vi "Main.vi"(8 "error in (no error)":errorcluster, 11 "GalvoBase in":refnum<class "ImagingModeSPIM.lvclass">) -> (0 "error out":errorcluster, 3 "component":refnum<class "ImagingModeSPIM.lvclass">)   [LabVIEW 2012, in "ImagingModeSPIM.lvclass"]
doc: "Main VI of the component."
uses:
  ImagingModeSPIM.lvclass
  Controls/waveform_enum.ctl
  ImagingModeSPIM.lvclass/ImagingModeSPIM.ctl
  <vilib>/Distrio/Murmex/InitialiseMessage/InitialiseMessage.lvclass
  <vilib>/Distrio/Murmex/TerminateMessage/TerminateMessage.lvclass
  <vilib>/Distrio/Murmex/ConfigureMessage/ConfigureMessage.lvclass
  <vilib>/Distrio/Murmex/StopMessage/StopMessage.lvclass
  <vilib>/Distrio/Murmex/StartMessage/run mode enum.ctl
  <vilib>/Distrio/Murmex/StartMessage/StartMessage.lvclass
  <vilib>/Distrio/Murmex/Murmex/update_cluster.ctl
  <vilib>/Distrio/Murmex/Murmex/Set configure at initialise.vi
  <vilib>/Distrio/Murmex/Murmex/Set VI reference.vi
  <vilib>/Distrio/Murmex/Murmex/Get ID.vi
  <vilib>/Distrio/Murmex/Murmex/Set relay start stop to observers.vi
  <vilib>/Distrio/Murmex/Murmex/Set log reference.vi
  <vilib>/Distrio/Murmex/Murmex/Set license required.vi
  <vilib>/Distrio/Murmex/StartMessage/Set run mode.vi
  <vilib>/Distrio/Murmex/Murmex/Murmex.lvclass
panel:
  in  "button::quit":bool
  in  "button:start_finite":bool
  in  "button:start_free-run":bool
  in  "button::configure":bool
  in  "Tab Control":T1(tab)
  in  "Phase 2":dbl[unit] caption="phase" min=-6.283185307179586 max=6.283185307179586 step=0.0017453292519943296
  in  "Offset 2":dbl[unit] caption="offset" min=-5.0 max=5.0 step=0.01
  in  "Amplitude 2":dbl[unit]=1.0 caption="amplitude" min=0.0 max=5.0 step=0.01
  in  "Phase 1":dbl[unit] caption="phase" min=-6.283185307179586 max=6.283185307179586 step=0.0017453292519943296
  in  "shape":T2
  in  "Offset 1":dbl[unit] caption="offset" min=-5.0 max=5.0 step=0.01
  in  "Amplitude 1":dbl[unit]=1.0 caption="amplitude" min=0.0 max=5.0 step=0.01
  in  "frame time":dbl[unit]=100.0
  in  "frames":i32=1
  in  "v lines":i32=2048 min=4 max=2048 step=4
  in  "digital pulses":i32=2 min=0 max=20 step=2
  in  "digital ratio":dbl(knob)=0.5 min=0.0 max=1.0 step=0.02 scale=0.0..1.0
  out "log":string
  in  "ID":string="spim"
  out "terminate?":bool=TRUE
  # "galvo 1"
  # "galvo 2"
  # "ImagingModeSPIM\n\nDeveloped by:\n\nMarcel van 't Hoff PhD, \nMarie Caroline Muellenbroich PhD, \nLudovico Silvestri PhD,\n   University of Florence, 2014"
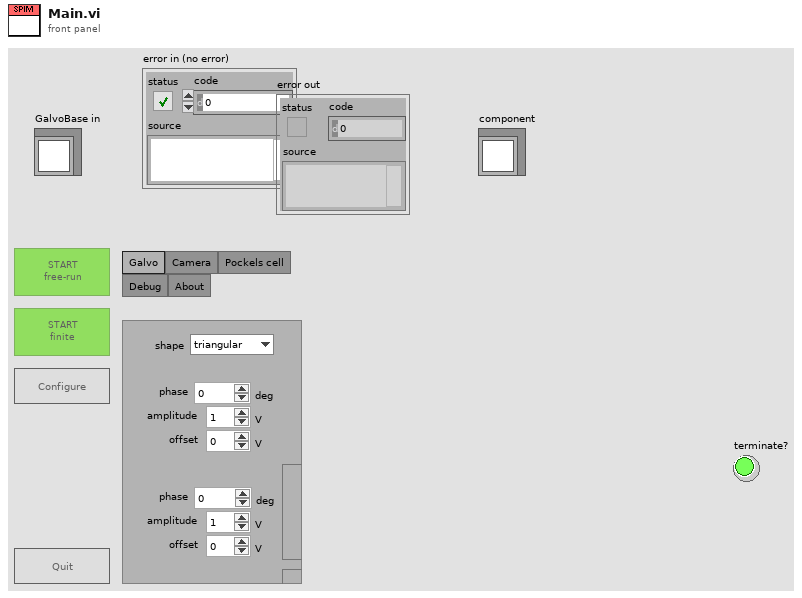
[diagram p1: front panel]
types:
  T1 = enum32{"Galvo", "Camera", "Pockels cell", "Debug", "About"}
  T2 = typedef "ImagingModeSPIM.lvclass/waveform_enum.ctl" = enum16{"triangular", "sawtooth", "sinusodial"}
  T3 = enum8{"Enabled", "Disabled", "Disabled and Grayed Out"}
  T4 = typedef "Murmex.lvlib/StartMessage.lvclass/run mode enum.ctl" = enum16{"infinite", "finite"}
  T5 = typedef "Murmex.lvlib/Murmex.lvclass/update_cluster.ctl" = cluster{"target ID":string, "key chains":string[], "values":variant[]}
  T6 = typedef "Murmex.lvlib/Murmex.lvclass/command_enum.ctl" = enum16{"null", "initialise", "reset", "terminate", "acknowledge", "update", "inspect", "inform", "proceed", "start", "stop", "fetch", "configure", "generic"}
  T7 = typedef "Murmex.lvlib/Murmex.lvclass/Event type enumerations.ctl" = enum16{"before", "after"}
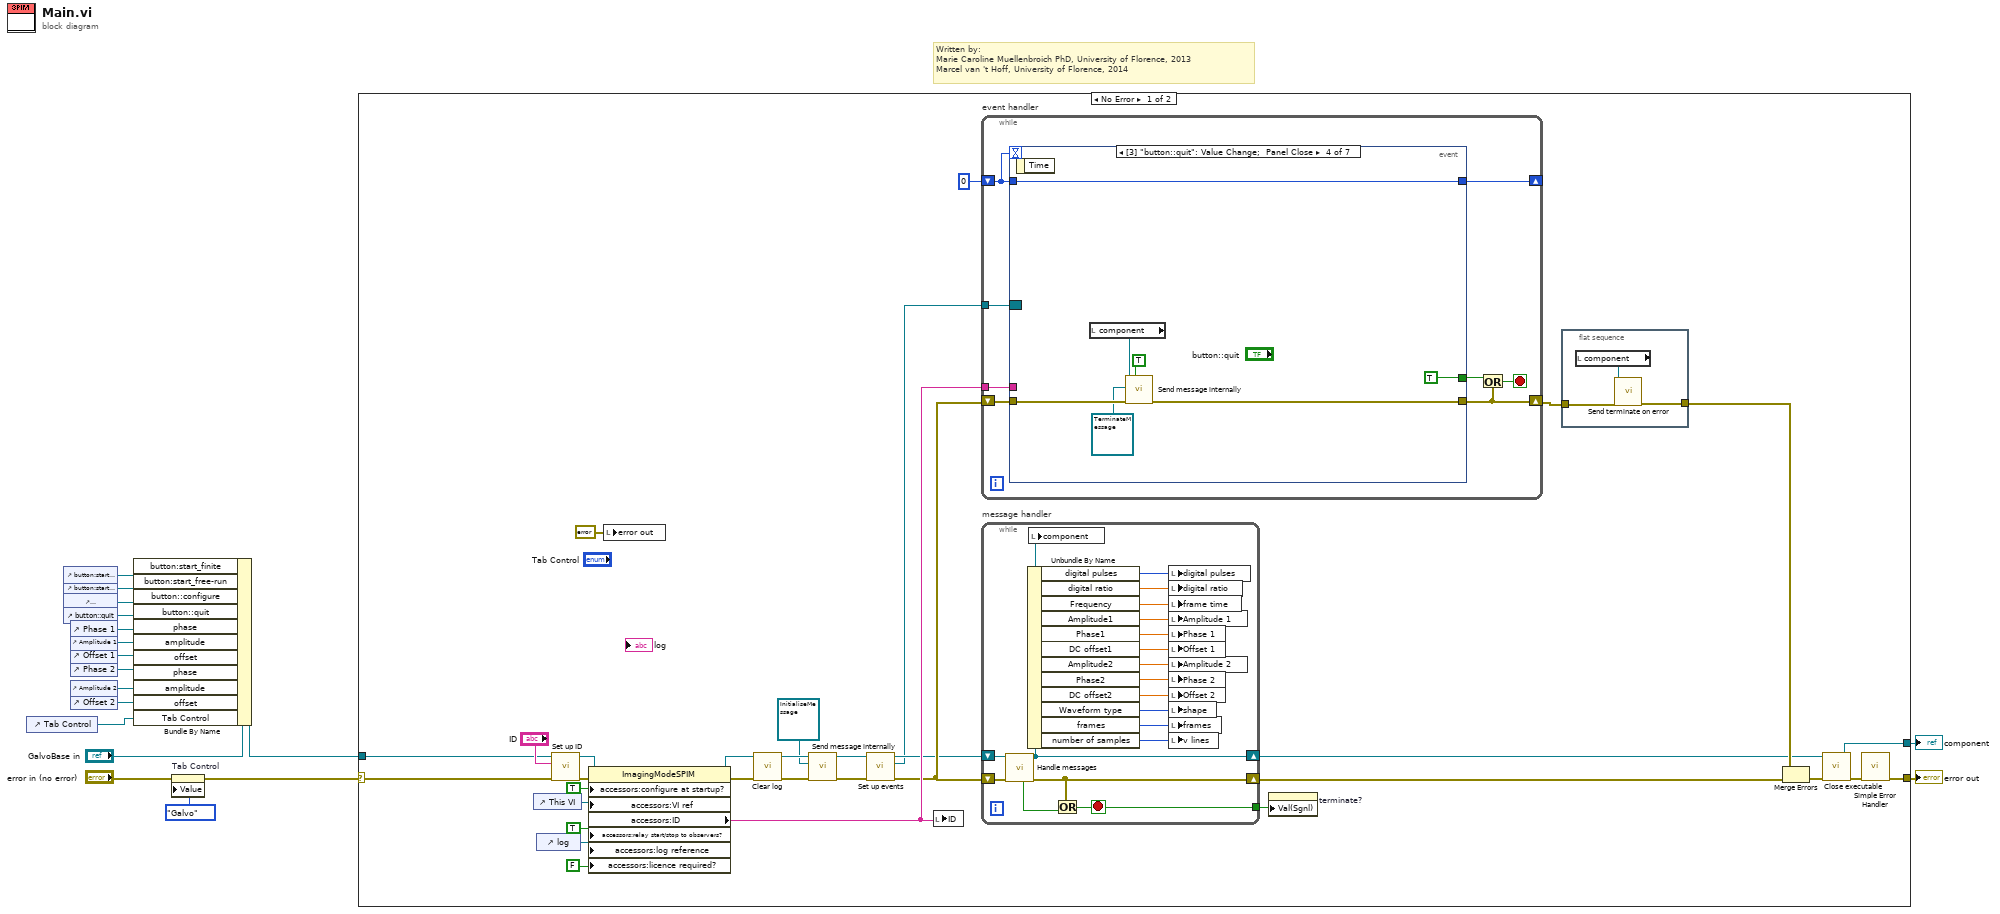
[diagram p0: block diagram]
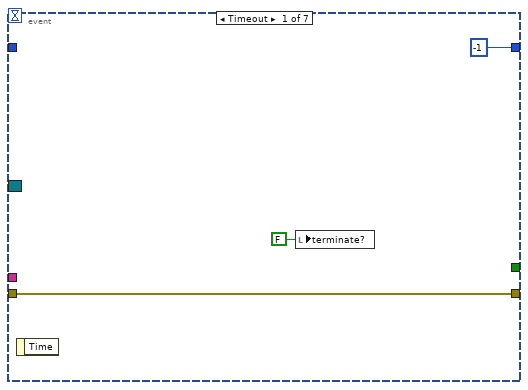
[diagram p2: hidden frame]
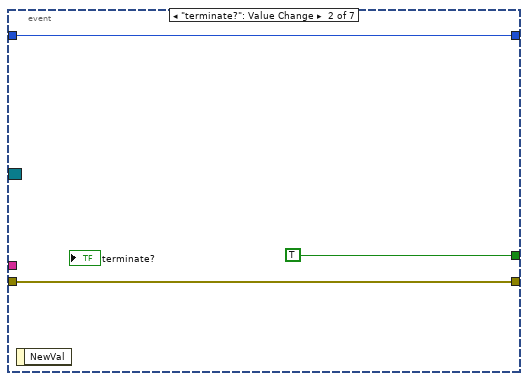
[diagram p3: hidden frame]
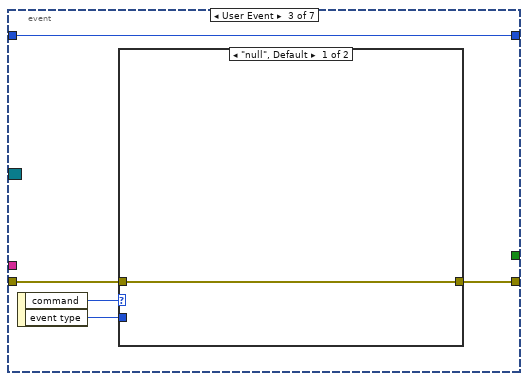
[diagram p4: hidden frame]
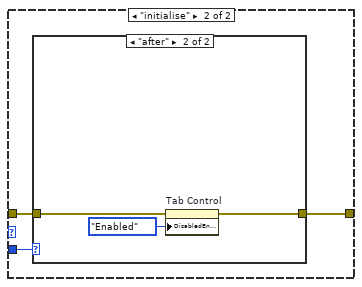
[diagram p5: hidden frame]
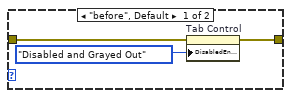
[diagram p6: hidden frame]
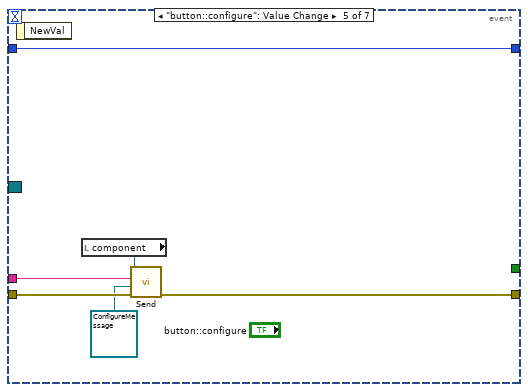
[diagram p7: hidden frame]
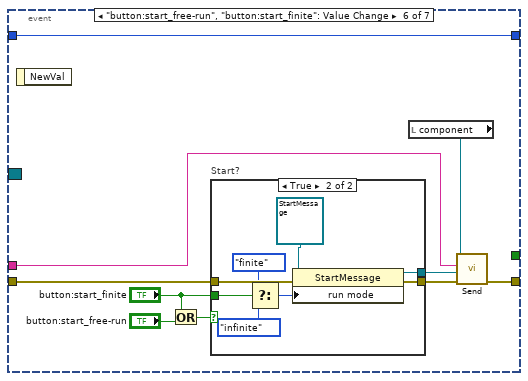
[diagram p8: hidden frame]
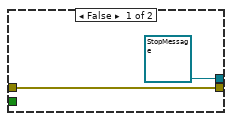
[diagram p9: hidden frame]
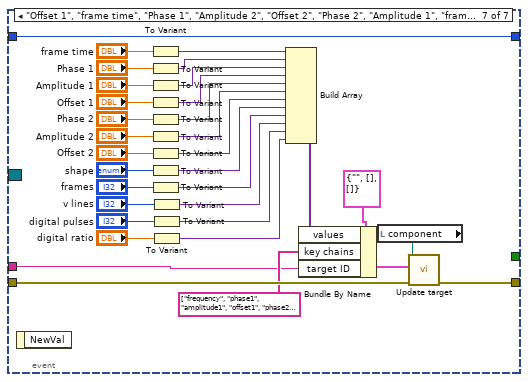
[diagram p10: hidden frame]
diagram:
  # "Written by:\nMarie Caroline Muellenbroich PhD, University of Florence, 2013 \nMarcel van 't Hoff, University of Florence, 2014"
  n1 = control-ref of="Tab Control"() -> (w3:refnum<vi>)
  n2 = control-ref of="button:start_finite"() -> (w15:refnum<vi>)
  n3 = control-ref of="button:start_free-run"() -> (w12:refnum<vi>)
  n4 = control-ref of="button::configure"() -> (w13:refnum<vi>)
  n5 = control-ref of="button::quit"() -> (w14:refnum<vi>)
  n6 = control-ref of="Phase 1"() -> (w11:refnum<vi>)
  n7 = control-ref of="Amplitude 1"() -> (w10:refnum<vi>)
  n8 = control-ref of="Offset 1"() -> (w9:refnum<vi>)
  n9 = control-ref of="Phase 2"() -> (w8:refnum<vi>)
  n10 = control-ref of="Amplitude 2"() -> (w7:refnum<vi>)
  n11 = control-ref of="Offset 2"() -> (w6:refnum<vi>)
  n12 = Bundle By Name(cluster="GalvoBase in", "button:start_finite"=w15, "button:start_free-run"=w12, "button::configure"=w13, "button::quit"=w14, "phase"=w11, "amplitude"=w10, "offset"=w9, "phase"=w8, "amplitude"=w7, "offset"=w6, "Tab Control"=w3) -> (w16:refnum<class "ImagingModeSPIM.lvclass">)
  n13 = property on="Tab Control" class="TabCtl (strict)"(error in="error in (no error)", "Value"=T1."Galvo" ("Tab Control")) -> (error out=w1:errorcluster)  [unwired: 1 in, 1 out]
  n14 = case shown="No Error" w1 {
    selector: w1 -> [w24 w167]
    tunnel: [w50 w167] -> w18
    tunnel: w16 -> [w32 w168]
    tunnel: [w49 w168] -> w2
    frame No Error {
      n15 = control-ref of="This VI"() -> (w47:refnum<vi>)
      n16 = control-ref of="log"() -> (w27:refnum<vi>)
      n17 = call <vilib>:"Set up ID.vi"("error in (no error)"=w24, "component ID"="ID", "MurmexBase in"=w32) -> ("error out"=w44:errorcluster, "MurmexBase out"=w45:refnum<class "ImagingModeSPIM.lvclass">)  [unwired: 6 in, 1 out]
      n18 = property class="ImagingModeSPIM"(reference=w45, error in=w44, "accessors:configure at startup?"=TRUE ("configure at startup?"), "accessors:VI ref"=w47, "accessors:relay start/stop to observers?"=TRUE ("relay start/stop to observers?"), "accessors:log reference"=w27, "accessors:licence required?"=FALSE ("licence required?")) -> (reference out=w29:refnum<class "ImagingModeSPIM.lvclass">, error out=w31:errorcluster, "accessors:ID"=w34:string)
      n19 = local write "error out"(errorcluster {"status"=FALSE, "code"=0, "source"=""} ("error out")) -> ()
      n20 = call <vilib>:"Clear log.vi"("error in (no error)"=w31, "MurmexBase in"=w29) -> ("error out"=w30:errorcluster, "MurmexBase out"=w28:refnum<class "ImagingModeSPIM.lvclass">)  [unwired: 8 in]
      n21 = call <vilib>:"Send message internally.vi"("error in (no error)"=w30, "Message"=refnum<class "InitialiseMessage.lvclass"> refnum ("Murmex.lvlib:InitialiseMessage"), "Murmex in"=w28) -> ("error out"=w23:errorcluster, "Murmex out"=w21:refnum<class "ImagingModeSPIM.lvclass">)  [unwired: 7 in]
      n22 = call <vilib>:"Set up events.vi"("error in (no error)"=w23, "MurmexBase in"=w21) -> ("error out"=w22:errorcluster, "Event Registration Refnum"=w19:refnum<event-registration>, "MurmexBase out"=w20:refnum<class "ImagingModeSPIM.lvclass">)  [unwired: 7 in]
      n23 = local write "ID"(w34) -> ()
      n24 = while "event handler" {
        shift-right: [w59] -> w42
        shift-left: w22 -> [w61]
        shift-right: [w55] -> _
        shift-left: 0 -> [w56]
        tunnel: w34 -> [w57]
        tunnel: w19 -> [w54]
        stop <- w58 stop-if-true
        n25 = event shown="[3] \"button::quit\": Value Change;  Panel Close" {
          selector: w54 -> [_ _ _ _ _ _ _]
          dyn-events: _ -> [_ _ _ _ _ _ _]
          timeout: w56 -> [_ _ _ _ _ _ _]
          tunnel: [w64 w67 w69 w89 w94 w99 w147] -> w59
          tunnel: w61 -> [w64 w67 w70 w88 w95 w104 w148]
          tunnel: [_ TRUE ("configure at startup?") _ TRUE ("configure at startup?") _ _ _] -> w60
          tunnel: w57 -> [_ _ _ _ w93 w96 w123]
          tunnel: w56 -> [_ w65 w68 w86 w92 w105 w134]
          tunnel: [-1 w65 w68 w86 w92 w105 w134] -> w55
          event Timeout {
            n26 = event-data() -> ()  [unwired: 1 in, 1 out]
            n27 = local write "terminate?"(FALSE ("terminate?")) -> ()
          }
          event "terminate?": Value Change {
            n28 = event-data() -> ()  [unwired: 1 in, 1 out]
          }
          event User Event {
            n29 = event-data() -> ("command"=w72:T6, "event type"=w71:T7)  [unwired: 1 in]
            n30 = case shown="\"null\", Default" w72 {
              tunnel: w71 -> [_ w76]
              tunnel: w70 -> [w73 w75]
              tunnel: [w73 w74] -> w69
              frame "null", Default {
              }
              frame "initialise" {
                n31 = case shown="\"after\"" w76 {
                  tunnel: w75 -> [w79 w82]
                  tunnel: [w78 w81] -> w74
                  frame "before", Default {
                    n32 = property on="Tab Control" class="TabCtl (strict)"(error in=w79, "DisabledEnum"=T3."Disabled and Grayed Out" ("Disabled")) -> (error out=w78:errorcluster)  [unwired: 1 in, 1 out]
                  }
                  frame "after" {
                    n33 = property on="Tab Control" class="TabCtl (strict)"(error in=w82, "DisabledEnum"=T3."Enabled" ("Disabled")) -> (error out=w81:errorcluster)  [unwired: 1 in, 1 out]
                  }
                }
              }
            }
          }
          event "button::quit": Value Change; Panel Close {
            n34 = event-data() -> ()  [unwired: 1 in, 1 out]
            n35 = local read "component"() -> (w85:refnum<class "ImagingModeSPIM.lvclass">)
            n36 = call <vilib>:"Send message internally.vi"("priority message? (F)"=TRUE, "error in (no error)"=w88, "Message"=refnum<class "TerminateMessage.lvclass"> refnum ("Murmex.lvlib:TerminateMessage"), "Murmex in"=w85) -> ("error out"=w89:errorcluster)  [unwired: 6 in, 1 out]
          }
          event "button::configure": Value Change {
            n37 = event-data() -> ()  [unwired: 1 in, 1 out]
            n38 = local read "component"() -> (w91:refnum<class "ImagingModeSPIM.lvclass">)
            n39 = call <vilib>:"Send.vi"("error in (no error)"=w95, "Message"=refnum<class "ConfigureMessage.lvclass"> refnum ("Murmex.lvlib:ConfigureMessage"), "recipient"=w93, "Murmex in"=w91) -> ("error out"=w94:errorcluster)  [unwired: 6 in, 1 out]
          }
          event "button:start_free-run", "button:start_finite": Value Change {
            n40 = event-data() -> ()  [unwired: 1 in, 1 out]
            n41 = Or(x="button:start_finite", y="button:start_free-run") -> (x .or. y?=w103:bool)
            n42 = case "Start?" shown="True" w103 {
              tunnel: w104 -> [w107 w115]
              tunnel: [w107 w110] -> w100
              tunnel: "button:start_finite" -> [_ w111]
              tunnel: [refnum<class "StopMessage.lvclass"> refnum ("Murmex.lvlib:StopMessage") w109] -> w97
              frame False {
              }
              frame True {
                n43 = Select(t=run_mode_enum."finite" ("run mode"), s=w111, f=run_mode_enum."infinite" ("run mode")) -> (s? t:f=w112:T4)
                n44 = property class="StartMessage"(reference=refnum<class "StartMessage.lvclass"> refnum ("Murmex.lvlib:StartMessage"), error in=w115, "run mode"=w112) -> (reference out=w109:refnum<class "StartMessage.lvclass">, error out=w110:errorcluster)
              }
            }
            n45 = local read "component"() -> (w98:refnum<class "ImagingModeSPIM.lvclass">)
            n46 = call <vilib>:"Send.vi"("error in (no error)"=w100, "Message"=w97, "recipient"=w96, "Murmex in"=w98) -> ("error out"=w99:errorcluster)  [unwired: 6 in, 1 out]
          }
          event "Offset 1", "frame time", "Phase 1", "Amplitude 2", "Offset 2", "Phase 2", "Amplitude 1", "frames", "v lines", "digital pulses", "digital ratio": Value Change {
            n47 = event-data() -> ()  [unwired: 1 in, 1 out]
            n48 = To Variant(anything="frame time") -> (Variant=w144:variant)
            n49 = To Variant(anything="Phase 1") -> (Variant=w141:variant)
            n50 = To Variant(anything="Amplitude 1") -> (Variant=w140:variant)
            n51 = To Variant(anything="Offset 1") -> (Variant=w139:variant)
            n52 = To Variant(anything="Phase 2") -> (Variant=w131:variant)
            n53 = To Variant(anything="Amplitude 2") -> (Variant=w130:variant)
            n54 = To Variant(anything="Offset 2") -> (Variant=w127:variant)
            n55 = To Variant(anything="shape") -> (Variant=w133:variant)
            n56 = To Variant(anything="frames") -> (Variant=w124:variant)
            n57 = To Variant(anything="v lines") -> (Variant=w120:variant)
            n58 = To Variant(anything="digital pulses") -> (Variant=w118:variant)
            n59 = To Variant(anything="digital ratio") -> (Variant=w117:variant)
            n60 = Build Array(w144, w141, w140, w139, w131, w130, w127, w133, w124, w120, w118, w117) -> (w143:variant[])
            n61 = Bundle By Name(cluster=T5 {"target ID"="", "key chains"=[], "values"=[]} ("update cluster"), "values"=w143, "key chains"=string[] ["frequency", "phase1", "amplitude1", "offset1", "phase2", "amplitude2", "offset2", "waveform_type", "frames", "lines", "digital_pulses", "digital_ratio"], "target ID"=w123) -> (w145:T5)
            n62 = local read "component"() -> (w122:refnum<class "ImagingModeSPIM.lvclass">)
            n63 = call <vilib>:"Update target.vi"("error in (no error)"=w148, "update cluster"=w145, "MurmexBase in"=w122) -> ("error out"=w147:errorcluster)  [unwired: 7 in, 1 out]
          }
        }
        n64 = Or(x=w60, y=w59) -> (x .or. y?=w58:bool)
      }
      n65 = while "message handler" {
        shift-right: [w150] -> w37
        shift-left: w20 -> [w165]
        shift-right: [w164] -> w40
        shift-left: w22 -> [w166]
        tunnel: [w162] -> w46
        stop <- w162 stop-if-true
        n66 = call <vilib>:"Handle messages.vi"("error in (no error)"=w166, "Murmex in"=w165) -> ("error out"=w164:errorcluster, "Murmex out"=w150:refnum<class "ImagingModeSPIM.lvclass">, "terminated?"=w163:bool)  [unwired: 7 in]
        n67 = Unbundle By Name(w150) -> ("digital pulses"=w151:i32, "digital ratio"=w152:dbl, "Frequency"=w149:dbl[unit], "Amplitude1"=w161:dbl[unit], "Phase1"=w159:dbl[unit], "DC offset1"=w157:dbl[unit], "Amplitude2"=w160:dbl[unit], "Phase2"=w158:dbl[unit], "DC offset2"=w156:dbl[unit], "Waveform type"=w155:T2, "frames"=w154:i32, "number of samples"=w153:i32)
        n68 = local write "component"(w150) -> ()
        n69 = Or(x=w164, y=w163) -> (x .or. y?=w162:bool)
        n70 = local write "digital pulses"(w151) -> ()
        n71 = local write "digital ratio"(w152) -> ()
        n72 = local write "frame time"(w149) -> ()
        n73 = local write "Amplitude 1"(w161) -> ()
        n74 = local write "Phase 1"(w159) -> ()
        n75 = local write "Offset 1"(w157) -> ()
        n76 = local write "Amplitude 2"(w160) -> ()
        n77 = local write "Phase 2"(w158) -> ()
        n78 = local write "Offset 2"(w156) -> ()
        n79 = local write "shape"(w155) -> ()
        n80 = local write "frames"(w154) -> ()
        n81 = local write "v lines"(w153) -> ()
      }
      n82 = property on="terminate?" class="Bool (strict)"("Val(Sgnl)"=w46) -> ()  [unwired: 2 in, 2 out]
      n83 = flat-sequence {
        tunnel: w42 -> [w53]
        tunnel: [w51] -> w41
        frame #0 {
          n84 = local read "component"() -> (w52:refnum<class "ImagingModeSPIM.lvclass">)
          n85 = call <vilib>:"Send terminate on error.vi"("error in (no error)"=w53, "Murmex in"=w52) -> ("error out"=w51:errorcluster)  [unwired: 8 in, 1 out]
        }
      }
      n86 = Merge Errors(w41, w40) -> (w39:errorcluster)
      n87 = call <vilib>:"Close executable.vi"("error in (no error)"=w39, "MurmexBase in"=w37) -> ("error out"=w38:errorcluster, "MurmexBase out"=w49:refnum<class "ImagingModeSPIM.lvclass">)  [unwired: 8 in]
      n88 = call <vilib>:"Simple Error Handler.vi"("error in (no error)"=w38) -> ("error out"=w50:errorcluster)  [unwired: 4 in, 4 out]
    }
    frame Error {
    }
  }
  "error out" <- w18
  "component" <- w2
